vi "PathPlanner_CommandExecute.vi"(9 "command":T4, 10 "Execute":bool=TRUE, 11 "in Timer":T1 {"Accumulated TIme" format="%13.5p"; "StartTime" format="%13.5p"}) -> (0 "CurrentTImer":dbl, 2 "Expired":bool, 3 "out Timer":T1 {"Accumulated TIme" format="%13.5p"; "StartTime" format="%13.5p"})   [LabVIEW 2023]
uses:
  <vilib>/Rock Robotics/WPI/ThirdParty/MJansen/PathPlanner/ENum/PathPlanner_CommandUtilType_ENUM.ctl
  <vilib>/Rock Robotics/WPI/ThirdParty/JAS_Junk/TrajLib/TypeDef/TIMER.ctl
  <vilib>/Rock Robotics/WPI/ThirdParty/JAS_Junk/TrajLib/MedianFilter_New.vi
  <vilib>/Rock Robotics/WPI/ThirdParty/JAS_Junk/TrajLib/MedianFilter_ResetToValue.vi
  <vilib>/Rock Robotics/WPI/ThirdParty/JAS_Junk/TrajLib/MedianFilter_Calculate.vi
  <vilib>/Utility/semaphor.llb/Obtain Semaphore Reference.vi
  <vilib>/Rock Robotics/WPI/ThirdParty/JAS_Junk/TrajLib/Timer_Reset.vi
  <vilib>/Rock Robotics/WPI/ThirdParty/JAS_Junk/TrajLib/Trajectory_Library.lvlib
  <vilib>/Rock Robotics/WPI/ThirdParty/MJansen/PathPlanner/PathPlanner24.lvlib
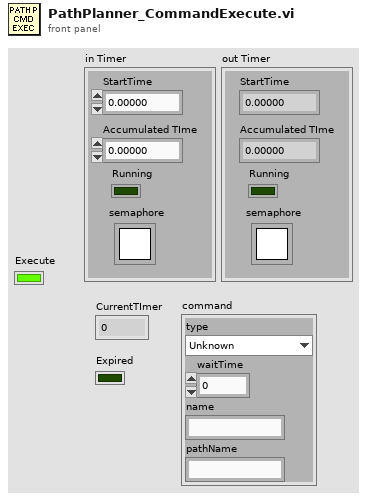
[diagram p1: front panel]
types:
  T1 = typedef "Trajectory_Library.lvlib/TIMER.ctl" = cluster{"StartTime":dbl, "Accumulated TIme":dbl, "Running":bool, "semaphore":T2}
  T2 = typedef "Semaphore RefNum" = refnum<k1>
  T3 = typedef "PathPlanner24.lvlib/PathPlanner_CommandUtilType_ENUM.ctl" = enum16{"Unknown", "Wait", "Named", "Path", "Sequential", "Parallel", "Race", "Deadline"}
  T4 = cluster{"type":T3, "waitTime":dbl, "name":string, "pathName":string}
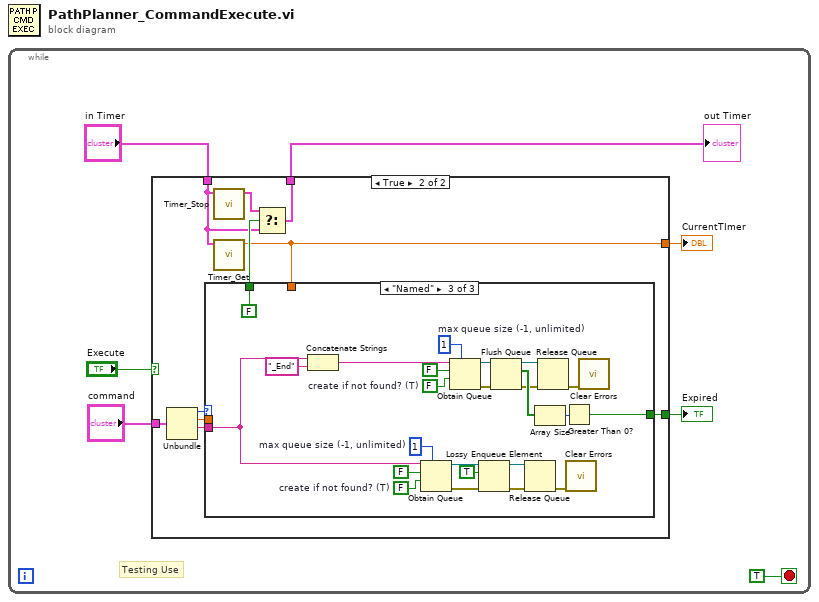
[diagram p0: block diagram]
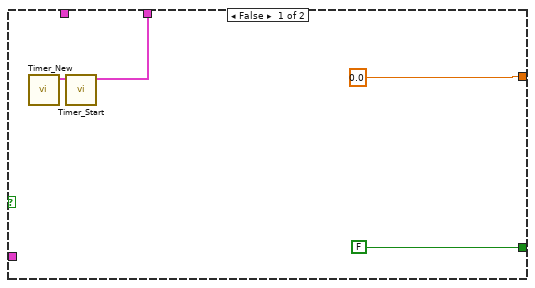
[diagram p2: hidden frame]
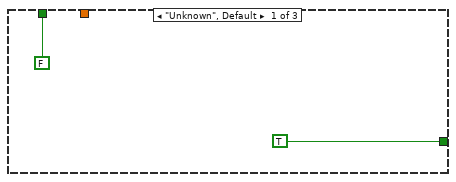
[diagram p3: hidden frame]
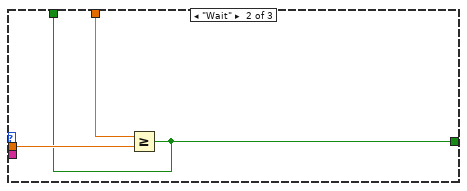
[diagram p4: hidden frame]
diagram:
  n1 = while {
    stop <- TRUE stop-if-true
    # "Testing Use"
    n2 = case shown="True" "Execute" {
      tunnel: "command" -> [_ w21]
      tunnel: [0.0 ("CurrentTImer") w12] -> w5
      tunnel: [FALSE w17] -> w4
      tunnel: "in Timer" -> [_ w14]
      tunnel: [w8 w13] -> w1
      frame False {
        n3 = call <vilib>:"Timer_New.vi"() -> ("TIMER"=w9:T1)  [unwired: 11 in]
        n4 = call <vilib>:"Timer_Start.vi"("in Timer"=w9) -> ("out Timer"=w8:T1)  [unwired: 10 in]
      }
      frame True {
        n5 = Unbundle(w21) -> ("type"=w20:T3, "waitTime"=w18:dbl, "name"=w19:string)  [unwired: 1 out]
        n6 = call <vilib>:"Timer_Stop.vi"("in Timer"=w14) -> ("out Timer"=w15:T1)  [unwired: 10 in]
        n7 = call <vilib>:"Timer_Get.vi"("TIMER"=w14) -> ("CurrentTImer"=w12:dbl)  [unwired: 10 in]
        n8 = case shown="\"Named\"" w20 {
          tunnel: w19 -> [_ _ w42]
          tunnel: w18 -> [_ w26 _]
          tunnel: [FALSE w24 FALSE] -> w16
          tunnel: w12 -> [_ w25 _]
          tunnel: [TRUE w24 w27] -> w17
          frame "Unknown", Default {
          }
          frame "Wait" {
            n9 = Greater Or Equal?(x=w25, y=w26) -> (x >= y?=w24:bool)
          }
          frame "Named" {
            w35 = FALSE  # create if not found? (T)
            w34 = 1  # max queue size (-1, unlimited)
            w45 = FALSE  # create if not found? (T)
            w44 = 1  # max queue size (-1, unlimited)
            n10 = Concatenate Strings(w42, "_End" ("string")) -> (w28:string)
            n11 = Obtain Queue(max queue size (-1, unlimited)=w44, name (unnamed)=w42, element data type=FALSE, create if not found? (T)=w45) -> (queue out=w48:refnum<queue>, error out=w49:errorcluster)  [unwired: 1 in, 1 out]
            n12 = Obtain Queue(max queue size (-1, unlimited)=w34, name (unnamed)=w28, element data type=FALSE, create if not found? (T)=w35) -> (queue out=w32:refnum<queue>, error out=w31:errorcluster)  [unwired: 1 in, 1 out]
            n13 = Lossy Enqueue Element(queue=w48, element=TRUE, error in (no error)=w49) -> (queue out=w39:refnum<queue>, error out=w41:errorcluster)  [unwired: 2 out]
            n14 = Flush Queue(queue=w32, error in (no error)=w31) -> (queue out=w30:refnum<queue>, remaining elements=w37:bool[], error out=w29:errorcluster)
            n15 = Release Queue(queue=w39, error in (no error)=w41) -> (error out=w40:errorcluster)  [unwired: 1 in, 2 out]
            n16 = Array Size(array=w37) -> (size(s)=w38:i32)
            n17 = Release Queue(queue=w30, error in (no error)=w29) -> (error out=w33:errorcluster)  [unwired: 1 in, 2 out]
            n18 = Greater Than 0?(x=w38) -> (x > 0?=w27:bool)
            n19 = call <vilib>:"Clear Errors.vi"("error in (no error)"=w40) -> ()  [unwired: 5 in, 2 out]
            n20 = call <vilib>:"Clear Errors.vi"("error in (no error)"=w33) -> ()  [unwired: 5 in, 2 out]
          }
        }
        n21 = Select(t=w15, s=w16, f=w14) -> (s? t:f=w13:T1)
      }
    }
    "CurrentTImer" <- w5
    "Expired" <- w4
    "out Timer" <- w1
  }
